vi "GlobalAT_SigGen.vi"() -> ()   [LabVIEW 2018]
panel:
  in  "MaxSamples":u16
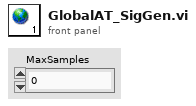
[diagram p1: front panel]
diagram:
